vi "get hdf device list swig.vi"(9 "nDevices":i32, 10 "monitor_ids":T1, 11 "file":string) -> (1 "nDevices out":i32, 2 "monitor_ids out":T1, 3 "file out":string, 5 "function return":i32)   [LabVIEW 2019, in "apdm.lvlib"]
doc: "APDM_EXPORT int apdm_get_hdf_device_list_swig(char *file, apdm_case_id_t *monitor_ids, int *nDevices);"
uses:
  apdm.lvlib
  Lee Lab/CP FES Walking 2018/Code/Working/LabVIEW/apdm.dll
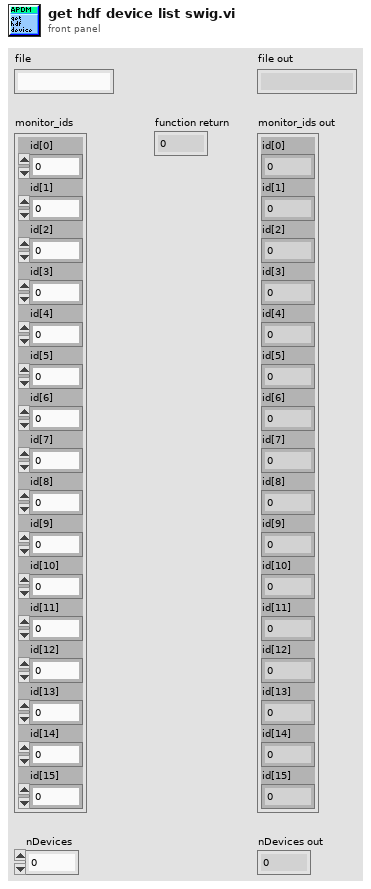
[diagram p1: front panel]
types:
  T1 = cluster{"id[0]":i8, "id[1]":i8, "id[2]":i8, "id[3]":i8, "id[4]":i8, "id[5]":i8, "id[6]":i8, "id[7]":i8, "id[8]":i8, "id[9]":i8, "id[10]":i8, "id[11]":i8, "id[12]":i8, "id[13]":i8, "id[14]":i8, "id[15]":i8}
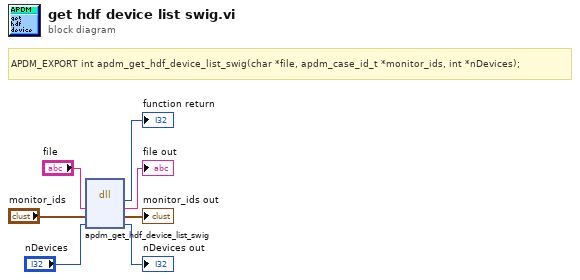
[diagram p0: block diagram]
diagram:
  # "APDM_EXPORT\tint apdm_get_hdf_device_list_swig(char *file, apdm_case_id_t *monitor_ids, int *nDevices);"
  n1 = dll-call lib="C:/Users/jfalesi/Dropbox/Lee Lab/CP FES Walking 2018/Code/Working/LabVIEW/apdm.*" fn="apdm_get_hdf_device_list_swig"("file"="file", "monitor_ids"="monitor_ids", "nDevices"="nDevices") -> (→"function return":i32, "file"=→"file out":string, "monitor_ids"=→"monitor_ids out":T1, "nDevices"=→"nDevices out":i32)  [unwired: 3 in, 2 out]
